vi "PWM Output Preview Gen.vi"(6 "Invert":bool, 9 "Low Level":dbl, 10 "High Level":dbl=1.0, 11 "Duty Cycle (4-96%)":dbl=20.0) -> (3 "Output Array":dbl[](array[numeric]))   [LabVIEW 2021]
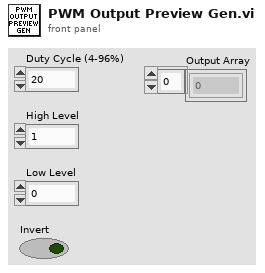
[diagram p1: front panel]
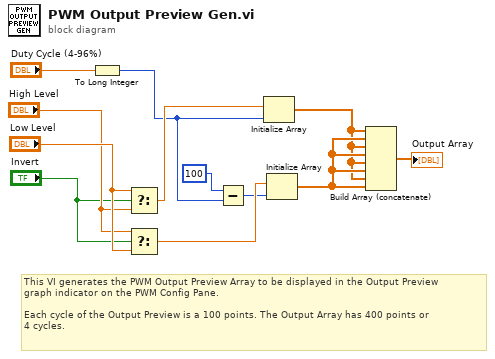
[diagram p0: block diagram]
diagram:
  # "This VI generates the PWM Output Preview Array to be displayed in the Output Preview \ngraph indicator on the PWM Config Pane.\n\nEach cycle of the Output Preview is a 100 points. The Output Array has 400 points or\n4 cycles."
  n1 = To Long Integer(number="Duty Cycle (4-96%)") -> (32bit integer=w5:i32)
  n2 = Select(t="Low Level", s="Invert", f="High Level") -> (s? t:f=w10:dbl)
  n3 = Select(t="High Level", s="Invert", f="Low Level") -> (s? t:f=w12:dbl)
  n4 = Subtract(x=100, y=w5) -> (x-y=w7:i32)
  n5 = Initialize Array(w10, w5) -> (w2:dbl[])
  n6 = Initialize Array(w12, w7) -> (w3:dbl[])
  n7 = Build Array (concatenate)(w2, w3, w2, w3, w2, w3, w2, w3) -> (→"Output Array":dbl[])
